vi "Set Image Properties.vi"(8 "error in":errorcluster, 11 "IMG_SRC in":refnum<class "IMG_SRC.lvclass">) -> (0 "error out":errorcluster, 3 "IMG_SRC out":refnum<class "IMG_SRC.lvclass">)   [LabVIEW 2018, in "IMG_SRC.lvlib" / "IMG_SRC.lvclass"]
uses:
  IMG_SRC.lvclass
  IMG_SRC.lvclass/IMG_SRC.ctl
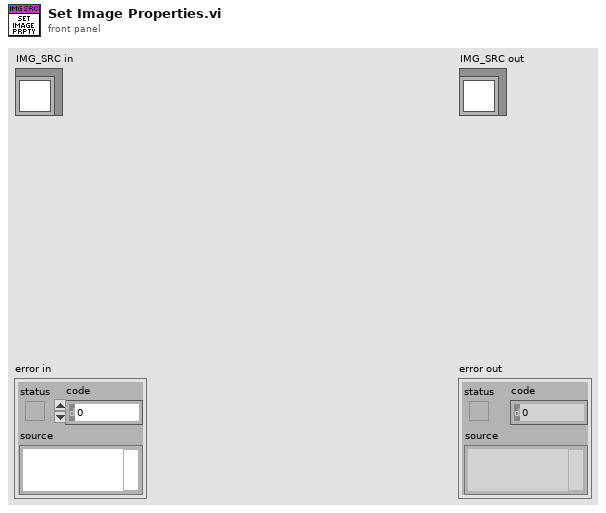
[diagram p1: front panel]
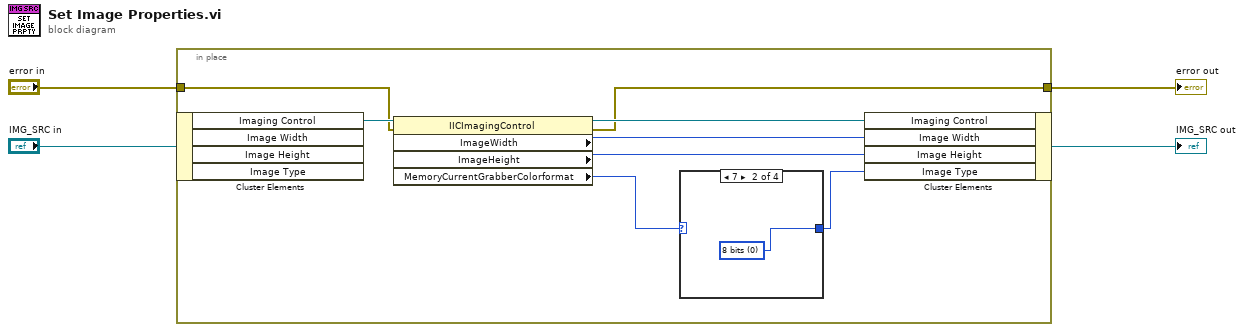
[diagram p0: block diagram]
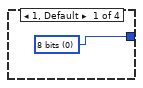
[diagram p2: hidden frame]
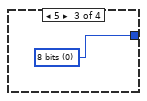
[diagram p3: hidden frame]
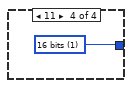
[diagram p4: hidden frame]
diagram:
  n1 = in-place {
    in-place-border: "error in" -> [w8]
    in-place-border: [w7] -> w2
    n2 = in-place-cluster #1("IMG_SRC in") -> ("Imaging Control"=w12:refnum<k7>)  [unwired: 3 out]
    n3 = property class="IICImagingControl"(reference=w12, error in=w8) -> (reference out=w11:refnum<k7>, error out=w7:errorcluster, "ImageWidth"=w10:i32, "ImageHeight"=w9:i32, "MemoryCurrentGrabberColorformat"=w5:i32)
    n4 = case shown="7" w5 {
      tunnel: [w13 w14 w15 w16] -> w6
      frame 1, Default {
        w13 = u32 0 items=["8 bits", "16 bits", "Float", "Complex", "RGB", "HSL"] ("Image Type")
      }
      frame 7 {
        w14 = u32 0 items=["8 bits", "16 bits", "Float", "Complex", "RGB", "HSL"] ("Image Type")
      }
      frame 5 {
        w15 = u32 0 items=["8 bits", "16 bits", "Float", "Complex", "RGB", "HSL"] ("Image Type")
      }
      frame 11 {
        w16 = u32 1 items=["8 bits", "16 bits", "Float", "Complex", "RGB", "HSL"] ("Image Type")
      }
    }
    n5 = in-place-cluster #1("Imaging Control"=w11, "Image Width"=w10, "Image Height"=w9, "Image Type"=w6) -> (→"IMG_SRC out":refnum<class "IMG_SRC.lvclass">)
  }
  "error out" <- w2
